vi "test2.vi"() -> ()   [LabVIEW 2011]
uses:
  <vilib>/Analysis/NI_AALBase.lvlib
panel:
  out "fit display":cluster{"X Values":dbl[], dbl[]}[](graph)
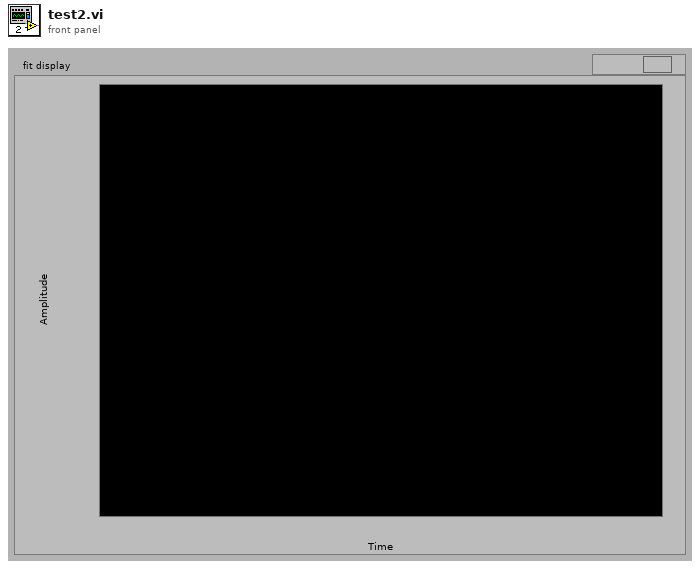
[diagram p1: front panel]
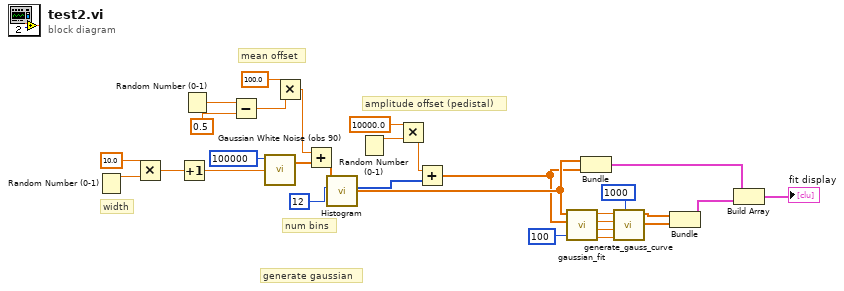
[diagram p0: block diagram]
diagram:
  # "num bins"
  # "width"
  # "amplitude offset (pedistal)"
  # "mean offset"
  # "generate gaussian"
  n1 = Random Number (0-1)() -> (number: 0 to 1=w13:dbl)
  n2 = Multiply(x=10.0, y=w13) -> (x*y=w12:dbl)
  n3 = Increment(x=w12) -> (x+1=w11:dbl)
  n4 = Random Number (0-1)() -> (number: 0 to 1=w6:dbl)
  n5 = Subtract(x=w6, y=0.5) -> (x-y=w4:dbl)
  n6 = call <vilib>:"Gaussian White Noise (obs 90).vi"("standard deviation"=w11, "samples"=100000) -> ("Gaussian noise pattern"=w8:dbl[])  [unwired: 1 in, 1 out]
  n7 = Multiply(x=100.0, y=w4) -> (x*y=w9:dbl)
  n8 = Add(x=w9, y=w8) -> (x+y=w7:dbl[])
  n9 = call <vilib>:"Histogram.vi"("intervals"=12, "X"=w7) -> ("X Values"=w20:dbl[], "Histogram: h(x)"=w16:i32[])  [unwired: 6 in, 2 out]
  n10 = Random Number (0-1)() -> (number: 0 to 1=w3:dbl)
  n11 = Multiply(x=10000.0, y=w3) -> (x*y=w1:dbl)
  n12 = Add(x=w1, y=w16) -> (x+y=w15:dbl[])
  n13 = call "gaussian_fit.vi"("Weights"=100, "Y Values"=w15, "X Values"=w20) -> ("offset"=w24:dbl, "StdDev"=w25:dbl, "Center"=w26:dbl, "Amplitude"=w27:dbl)  [unwired: 1 in, 2 out]
  n14 = Bundle("X Values"=w20, w15) -> (w19:cluster{"X Values":dbl[], dbl[]})  [unwired: 1 in]
  n15 = call "generate_gauss_curve.vi"("num points"=1000, "offset"=w24, "Spread"=w25, "Center"=w26, "Amplitude"=w27) -> ("Y Values"=w21:dbl[], "X Values"=w22:dbl[])  [unwired: 3 in]
  n16 = Bundle("X Values"=w22, "Y Values"=w21) -> (w18:cluster{"X Values":dbl[], "Y Values":dbl[]})  [unwired: 1 in]
  n17 = Build Array(w19, w18) -> (→"fit display":cluster{"X Values":dbl[], "Y Values":dbl[]}[])
